vi "load model plugin.vi"(7 "model name":string, 11 "error in (no error)":errorcluster) -> (4 "Model plugin":refnum<class "Abstract Model.lvclass">, 15 "error out":errorcluster)   [LabVIEW 2022 SP3]
uses:
  <vilib>/ErrorRing/Error Ring.xnode
  <vilib>/Utility/LVLibp/NI_PackedLibraryUtility.lvlib
  <vilib>/Utility/error.llb/Error Cluster From Error Code.vi
  Abstract Model/Abstract Model.lvlibp/Abstract Model.lvclass
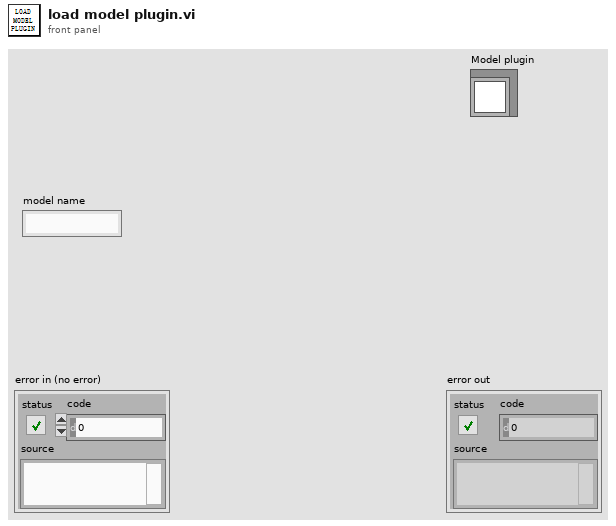
[diagram p1: front panel]
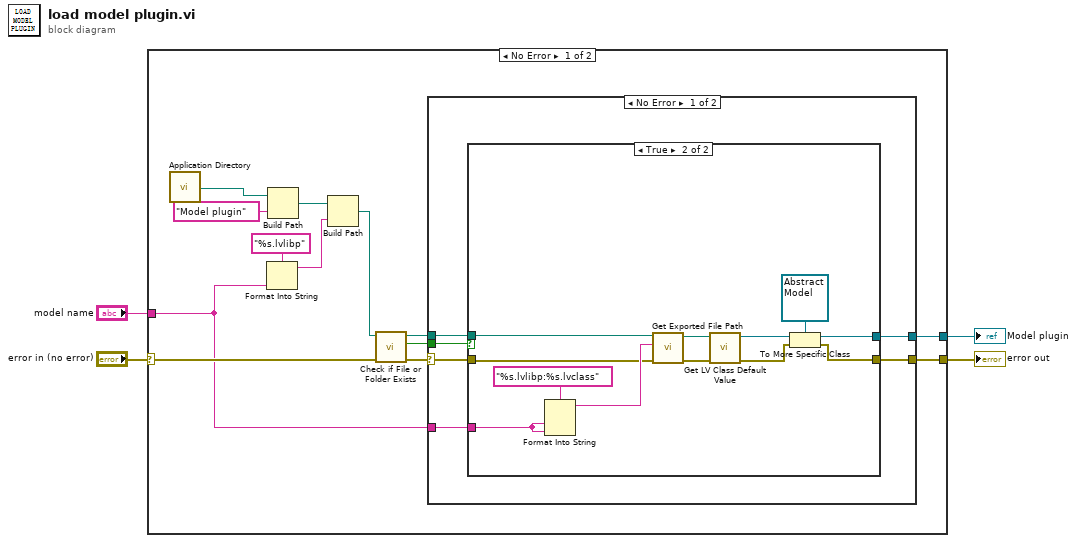
[diagram p0: block diagram]
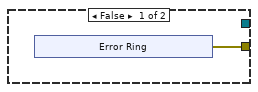
[diagram p2: hidden frame]
diagram:
  n1 = case shown="No Error" "error in (no error)" {
    selector: "error in (no error)" -> [w10 w43]
    tunnel: [w15 w43] -> w4
    tunnel: [w14 _] -> w1
    tunnel: "model name" -> [w5 _]
    frame No Error {
      n2 = call <vilib>:"Application Directory.vi"() -> ("Application Directory"=w17:path)
      n3 = Format Into String(format string="%s.lvlibp", w5) -> (resulting string=w11:string)  [unwired: 2 in, 1 out]
      n4 = Build Path(base path=w17, name or relative path="Model plugin") -> (appended path=w13:path)
      n5 = Build Path(base path=w13, name or relative path=w11) -> (appended path=w9:path)
      n6 = call <vilib>:"Check if File or Folder Exists.vi"("error in (no error)"=w10, "path"=w9) -> ("error out"=w8:errorcluster, "file or folder exists?"=w7:bool, "dup path"=w6:path)  [unwired: 7 in]
      n7 = case shown="No Error" w8 {
        selector: w8 -> [w23 w42]
        tunnel: [w22 w42] -> w15
        tunnel: [w21 _] -> w14
        tunnel: w7 -> [w20 _]
        tunnel: w6 -> [w18 _]
        tunnel: w5 -> [w19 _]
        frame No Error {
          n8 = case shown="True" w20 {
            tunnel: w23 -> [_ w39]
            tunnel: [w24 w34] -> w22
            tunnel: [_ w33] -> w21
            tunnel: w19 -> [_ w31]
            tunnel: w18 -> [_ w32]
            frame False {
              n9 = xnode "Error Ring"() -> ("error out"=w24:errorcluster)
            }
            frame True {
              n10 = Format Into String(format string="%s.lvlibp:%s.lvclass", w31, w31) -> (resulting string=w40:string)  [unwired: 2 in, 1 out]
              n11 = call <vilib>:"Get Exported File Path.vi"("error in (no error)"=w39, "qualified name"=w40, "packed library path"=w32) -> ("error out"=w38:errorcluster, "path"=w37:path)  [unwired: 7 in]
              n12 = call <vilib>:"Get LV Class Default Value.vi"("error in (no error)"=w38, "class path"=w37) -> ("error out"=w35:errorcluster, "object"=w36:refnum<class>)  [unwired: 8 in]
              n13 = To More Specific Class(target class=refnum<class "Abstract Model.lvclass"> refnum ("Abstract Model.lvlibp:Abstract Model.lvclass"), reference=w36, error in=w35) -> (specific class reference=w33:refnum<class "Abstract Model.lvclass">, error out=w34:errorcluster)
            }
          }
        }
        frame Error {
        }
      }
    }
    frame Error {
    }
  }
  "error out" <- w4
  "Model plugin" <- w1
